vi "Send Email using SMTP Client (tester).vi"() -> ()   [LabVIEW 2019]
doc: "Uses the SMTP Email Client to send an email to a standard or secure SMTP server."
uses:
  <vilib>/smtpClient/Set Message Text.vi
  <vilib>/smtpClient/LabVIEWSMTPClient.lvlib
panel:
  out "invalid recipients":string[](array[string])
  out "error out 2":errorcluster
  in  "Sender's Email Address":string
  in  "Message":string="Hopefully, sending alerts"
  in  "Subject":string="Testing the DrDAS"
  in  "To:":string="robert.raye@nrel.gov"
  in  "Password":string
  in  "Username":string
  in  "Port":string="587"
  in  "Outgoing Mail Server (SMTP)":string
  # "Overview: Connects to an SMTP Email Server, and sends one or more emails.\nRequirements: LabVIEW Full Development System\nInstructions:\n1. Run the VI.\n2. Configure the Outgoing Mail Server section, then click Configure Server.\n3. Specify the Compose Email content, then click Send Email.\n4. Click Stop to stop the VI."
  # "Outgoing Mail Server"
  # "Compose Email"
  # "Optional Parameters"
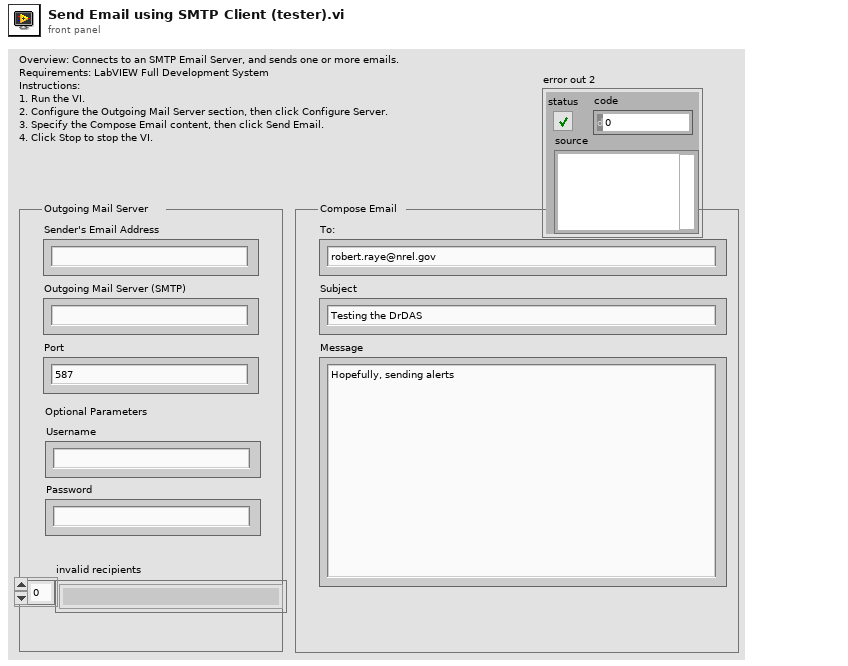
[diagram p1: front panel]
types:
  T1 = typedef "LabVIEWSMTPClient.lvlib/SmtpClientHandle.ctl" = refnum<k1>
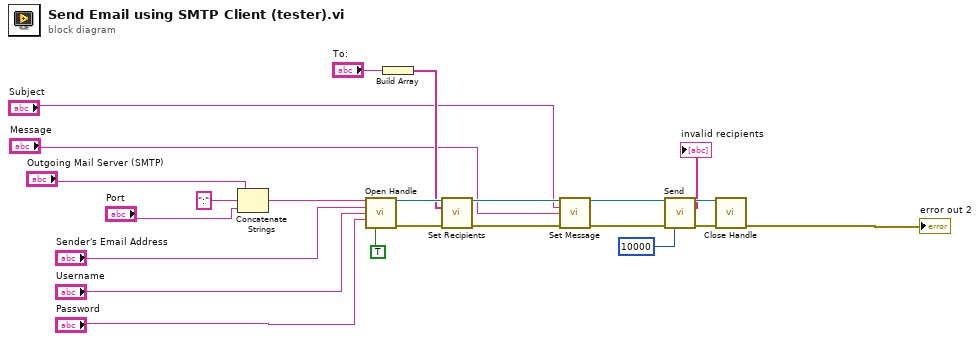
[diagram p0: block diagram]
diagram:
  n1 = Concatenate Strings("Outgoing Mail Server (SMTP)", ":" ("string"), "Port") -> (w11:string)
  n2 = call <vilib>:"Open Handle.vi"("server address"=w11, "from"="Sender's Email Address", "username"="Username", "password"="Password", "use TLS (false)"=TRUE ("Enable TLS")) -> ("handle out"=w19:T1, "error out"=w20:errorcluster)  [unwired: 9 in]
  n3 = Build Array("To:") -> (w8:string[])
  n4 = call <vilib>:"Set Recipients.vi"("handle in"=w19, "to"=w8, "error in (no error)"=w20) -> ("handle out"=w16:T1, "error out"=w17:errorcluster)  [unwired: 11 in]
  n5 = call-poly <vilib>:"Set Message.vi"("handle in"=w16, "subject"="Subject", "plain text message"="Message", "error in (no error)"=w17) -> ("handle out"=w14:T1, "error out"=w15:errorcluster)  [unwired: 10 in]
  n6 = call <vilib>:"Send.vi"("handle in"=w14, "error in (no error)"=w15, "timeout in ms (10000)"=10000 ("timeout in ms")) -> ("handle out"=w21:T1, "invalid recipients"=→"invalid recipients":string[], "error out"=w22:errorcluster)  [unwired: 10 in]
  n7 = call <vilib>:"Close Handle.vi"("handle in"=w21, "error in (no error)"=w22) -> ("error out"=→"error out 2":errorcluster)  [unwired: 12 in, 1 out]
